vi "Stop Working Thread.vi"(8 "error in (no error)":errorcluster, 9 "Operation":enum16{"Get", "Set"}(ring), 11 "Stop the working thread":bool) -> (0 "error out":errorcluster, 3 "Stop the working thread(out)":bool)   [LabVIEW 2017, in "WebServiceImporter.lvlib" / "Main Panel.lvlib" / "Progress.lvlib"]
uses:
  <vilib>/Platform/WebService/Main Panel/Pages/Progress/Progress.lvlib
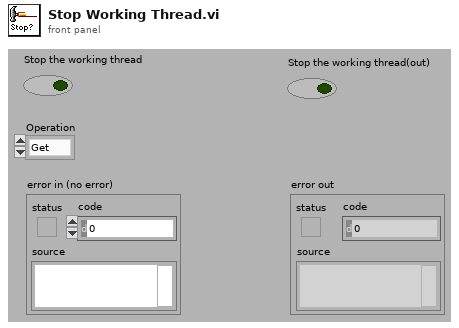
[diagram p1: front panel]
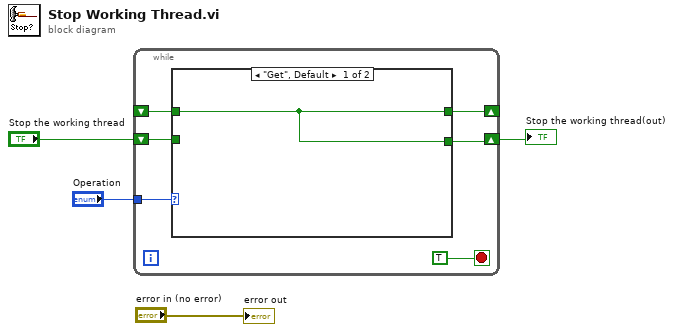
[diagram p0: block diagram]
diagram:
  n1 = while {
    tunnel: "Operation" -> [w10]
    shift-right: [w7] -> w2
    shift-left: "Stop the working thread" -> [w8]
    shift-right: [w6] -> _
    shift-left: _ -> [w5]
    stop <- TRUE stop-if-true
    n2 = case shown="\"Get\", Default" w10 {
      tunnel: [w11 w12] -> w7
      tunnel: w8 -> [_ w12]
      tunnel: [w11 w12] -> w6
      tunnel: w5 -> [w11 _]
      frame "Get", Default {
      }
      frame "Set" {
      }
    }
  }
  "Stop the working thread(out)" <- w2
  "error out" <- "error in (no error)"
